vi "NewSubArray.vi"(9 "Posit Array":T1[](array[typedef]), 11 "All Lines":T2) -> (1 "Array Length":i32, 2 "subarray":T1[](array[typedef]))   [LabVIEW 2014]
uses:
  Libraries/Map Data Folder/All-Lines.ctl
  Libraries/Map Data Folder/LineCluster.ctl
  Libraries/Map Data Folder/LineConnection.ctl
  Libraries/Contact Data/Position.ctl
  Libraries/Map Data Folder/Map Data.lvlib
  Libraries/Contact Data/Contact Data.lvlib
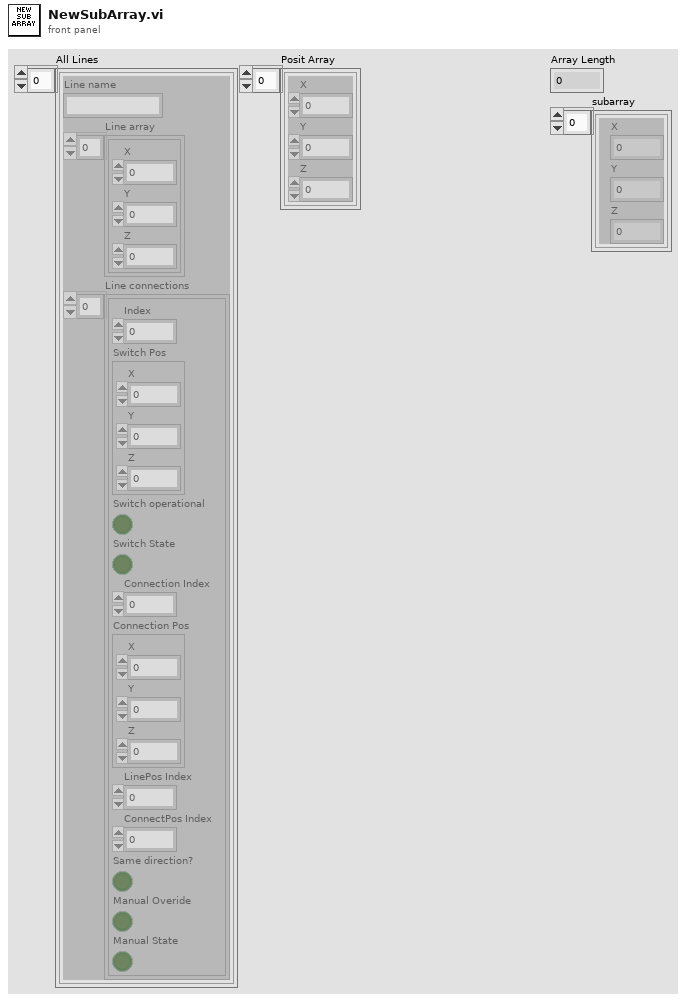
[diagram p1: front panel]
types:
  T1 = typedef "Contact Data.lvlib/Position.ctl" = cluster{"X":dbl, "Y":dbl, "Z":dbl}
  T2 = typedef "Map Data.lvlib/All-Lines.ctl" = T3[]
  T3 = typedef "Map Data.lvlib/LineCluster.ctl" = cluster{"Line name":string, "Line array":cluster{"X":dbl, "Y":dbl, "Z":dbl}[], "Line connections":T4[]}
  T4 = typedef "Map Data.lvlib/LineConnection.ctl" = cluster{"Index":i32, "Switch Pos":cluster{"X":dbl, "Y":dbl, "Z":dbl}, "Switch operational":bool, "Switch State":bool, "Connection Index":i32, "Connection Pos":cluster{"X":dbl, "Y":dbl, "Z":dbl}, "LinePos Index":i32, "ConnectPos Index":i32, "Same direction?":bool, "Manual Overide":bool, "Manual State":bool}
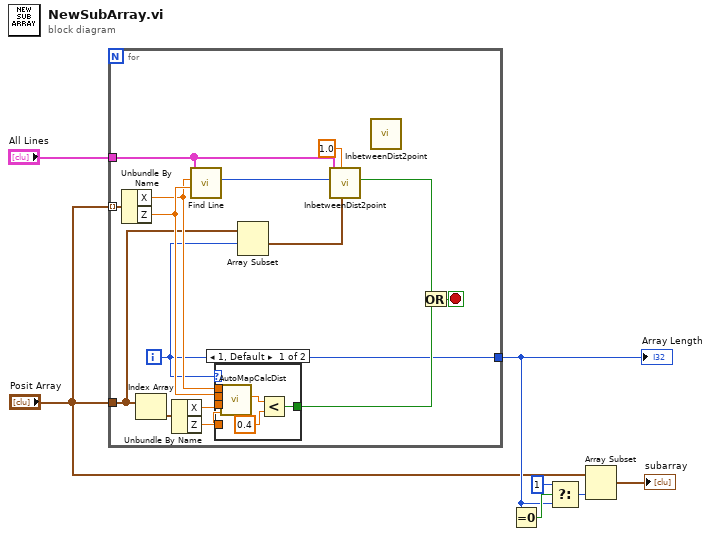
[diagram p0: block diagram]
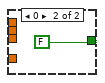
[diagram p2: hidden frame]
diagram:
  n1 = for {
    tunnel: "All Lines" -> [w19]
    tunnel: "Posit Array" -> [w20] mode=indexing
    tunnel: [w8] -> w3
    tunnel: "Posit Array" -> [w9]
    i -> [w8]
    stop <- w14 stop-if-true
    n2 = Unbundle By Name(w20) -> ("X"=w11:dbl, "Z"=w17:dbl)
    n3 = Index Array(array=w9) -> (element=w18:T1)  [unwired: 1 in]
    n4 = Unbundle By Name(w18) -> ("X"=w16:dbl, "Z"=w15:dbl)
    n5 = call "Find Line.vi"("Z"=w17, "X"=w11, "All Lines"=w19) -> ("Nearest Line"=w22:i32)  [unwired: 5 in, 3 out]
    n6 = case shown="1, Default" w8 {
      tunnel: w11 -> [w29 _]
      tunnel: w17 -> [w28 _]
      tunnel: w16 -> [w27 _]
      tunnel: w15 -> [w26 _]
      tunnel: [w24 FALSE] -> w13
      frame 1, Default {
        n7 = call "AutoMapCalcDist.vi"("Y2"=w26, "X2"=w27, "Y1"=w28, "X1"=w29) -> ("Distance"=w25:dbl)  [unwired: 7 in]
        n8 = Less?(x=w25, y=0.4) -> (x < y?=w24:bool)
      }
      frame 0 {
      }
    }
    n9 = Array Subset(array=w9, index=w8) -> (w10:T1[])  [unwired: 1 in]
    n10 = call "InbetweenDist2point.vi"("Posit Array"=w10, "Inbetween diff"=1.0, "Index"=w22, "All Lines"=w19) -> ("In range?"=w12:bool)  [unwired: 5 in, 2 out]
    n11 = call "InbetweenDist2point.vi"() -> ()  [unwired: 9 in, 3 out]
    n12 = Or(x=w12, y=w13) -> (x .or. y?=w14:bool)
  }
  "Array Length" <- w3
  n13 = Equal To 0?(x=w3) -> (x = 0?=w6:bool)
  n14 = Select(t=1, s=w6, f=w3) -> (s? t:f=w4:i32)
  n15 = Array Subset(array="Posit Array", length=w4) -> (→"subarray":T1[])  [unwired: 1 in]
